vi "DataProcess_RecreateProcessesFiles.vi"() -> ()   [LabVIEW 2016]
uses:
  ExpData/ExpData.lvclass
panel:
  out "Marked":bool
  out "Current":i32
  out "Total":i32
  in  "pattern":string
  in  "Output Path":path=path "E:/Dropbox (Lab)/C-ALEX/Experiments/Exp6-Stroke/clx_marked2"
  in  "Input Path":path=path "E:/Dropbox (Lab)/C-ALEX/Experiments/Exp6-Stroke/clx_marked"
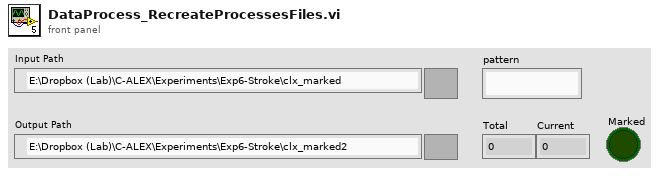
[diagram p1: front panel]
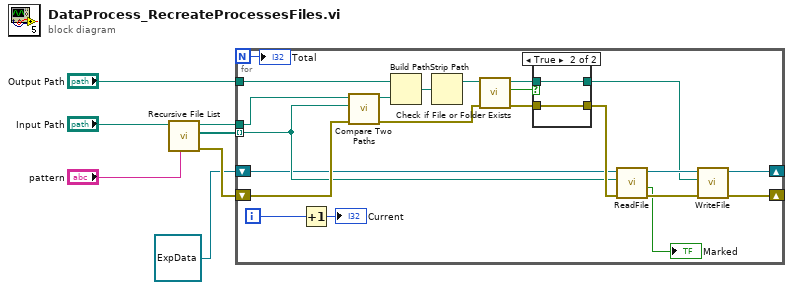
[diagram p0: block diagram]
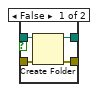
[diagram p2: hidden frame]
diagram:
  n1 = call <vilib>:"Recursive File List.vi"("pattern"="pattern", "Folder Path"="Input Path") -> ("error out"=w7:errorcluster, "All Files in Dir"=w6:path[], "dup Folder Path"=w3:path)  [unwired: 5 in, 2 out]
  n2 = for {
    N -> [w13]
    tunnel: w6 -> [w22] mode=indexing
    shift-right: [w27] -> _
    shift-left: w7 -> [w24]
    tunnel: "Output Path" -> [w21]
    tunnel: w3 -> [w23]
    shift-right: [w11] -> _
    shift-left: refnum<class "ExpData.lvclass"> refnum ("CarexData Out") -> [w10]
    i -> [w12]
    n3 = Increment(x=w12) -> (x+1=→"Current":i32)
    n4 = call <vilib>:"Compare Two Paths.vi"("error in (no error)"=w24, "Path 2"=w22, "Path 1"=w23) -> ("error out"=w16:errorcluster, "Relative Path from 1 to 2"=w20:path)  [unwired: 5 in, 2 out]
    n5 = Build Path(base path=w21, name or relative path=w20) -> (appended path=w19:path)
    n6 = Strip Path(path=w19) -> (stripped path=w18:path)  [unwired: 1 out]
    n7 = call <vilib>:"Check if File or Folder Exists.vi"("error in (no error)"=w16, "path"=w18) -> ("error out"=w15:errorcluster, "file or folder exists?"=w14:bool, "dup path"=w17:path)  [unwired: 7 in]
    n8 = case shown="True" w14 {
      tunnel: [w33 w34] -> w26
      tunnel: [w32 w35] -> w25
      tunnel: w17 -> [w31 w35]
      tunnel: w15 -> [w30 w34]
      frame False {
        n9 = Create Folder(path (use dialog)=w31, error in=w30) -> (created path=w32:path, error out=w33:errorcluster)  [unwired: 1 in, 1 out]
      }
      frame True {
      }
    }
    n10 = call "ReadFile.vi"("error in (no error)"=w26, "ExpData File Path"=w22, "ExpData In"=w10) -> ("error out"=w28:errorcluster, "Marked"=→"Marked":bool, "ExpData Out"=w29:refnum<class "ExpData.lvclass">)  [unwired: 5 in, 1 out]
    n11 = call "WriteFile.vi"("error in (no error)"=w28, "Output Path"=w25, "ExpData In"=w29) -> ("error out"=w27:errorcluster, "ExpData Out"=w11:refnum<class "ExpData.lvclass">)  [unwired: 6 in, 1 out]
    "Total" <- w13
  }
